vi "MAIN_camera_initialization_results.vi"(5 "error in":errorcluster, 8 "variant":variant) -> (0 "error out":errorcluster, 1 "Error":bool, 2 "Cooler status":bool, 3 "Real time image":T1, 4 "Total kinetic time (s)":sgl)   [LabVIEW 2015]
uses:
  <vilib>/vision/Image Controls.llb/IMAQ Image.ctl
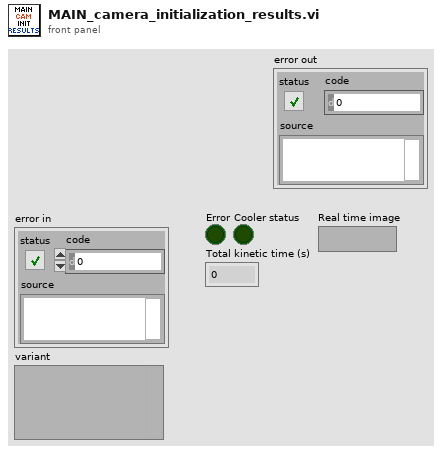
[diagram p1: front panel]
types:
  T1 = typedef "IMAQ Image.ctl" = refnum<image>
  T2 = cluster{"Total kinetic time (s)":sgl, "temperature":sgl, "coolerStatus":i32, "Error":bool, "Real time image":T1}
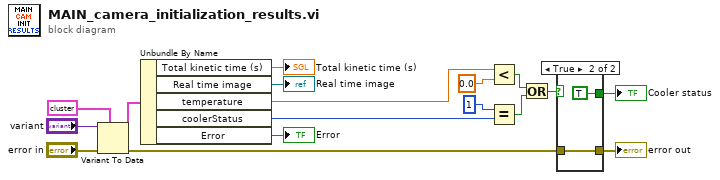
[diagram p0: block diagram]
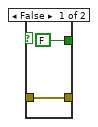
[diagram p2: hidden frame]
diagram:
  n1 = Variant To Data(error in="error in", type=T2 {"Total kinetic time (s)"=0.0, "temperature"=0.0, "coolerStatus"=0, "Error"=FALSE, "Real time image"=refnum}, Variant="variant") -> (data=w16:T2, error out=w7:errorcluster)
  n2 = Unbundle By Name(w16) -> ("Total kinetic time (s)"=→"Total kinetic time (s)":sgl, "Real time image"=→"Real time image":T1, "temperature"=w8:sgl, "coolerStatus"=w5:i32, "Error"=→"Error":bool)
  n3 = Less?(x=w8, y=sgl 0.0) -> (x < y?=w10:bool)
  n4 = Equal?(x=1, y=w5) -> (x = y?=w9:bool)
  n5 = Or(x=w10, y=w9) -> (x .or. y?=w13:bool)
  n6 = case shown="True" w13 {
    tunnel: w7 -> [w19 w21]
    tunnel: [w19 w21] -> w1
    tunnel: [FALSE TRUE] -> w4
    frame False {
    }
    frame True {
    }
  }
  "Cooler status" <- w4
  "error out" <- w1
